vi "获得取向.vi"(10 "角度输入":dbl[](array[numeric]), 11 "目标位置":dbl[](array[numeric])) -> (3 "取向输出":dbl[][](array[numeric]))   [LabVIEW 2017]
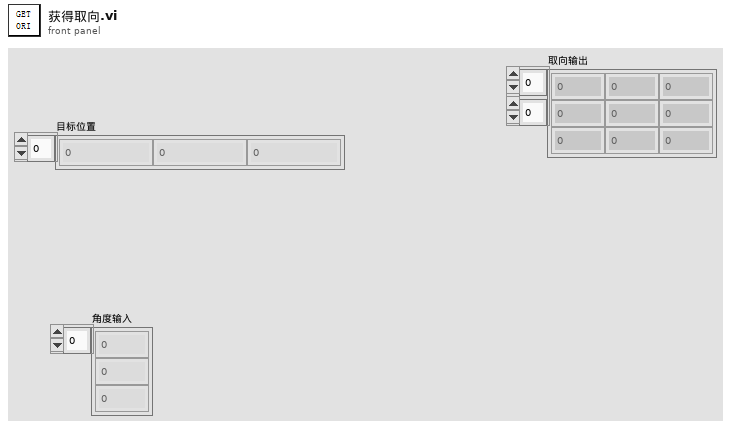
[diagram p1: front panel]
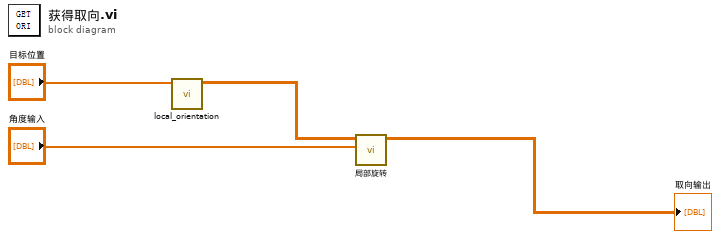
[diagram p0: block diagram]
diagram:
  n1 = call "local_orientation.vi"("目标位置"="目标位置") -> ("Array"=w4:dbl[][])  [unwired: 10 in]
  n2 = call "局部旋转.vi"("角度输入"="角度输入", "取向输入"=w4) -> ("取向输出"=→"取向输出":dbl[][])  [unwired: 9 in]
